vi "Simple Get Buffer.vi"(0 "remote file uri":string, 1 "username":string, 2 "password":string, 11 "error in (no error)":errorcluster) -> (4 "data":string, 15 "error out":errorcluster)   [LabVIEW 2017, in "NI_WebDAV.lvlib"]
doc: "Returns a file or multiple files or the raw binary contents of a file or multiple files from a remote WebDAV server or target. You must manually select the polymorphic instance you want to use."
uses:
  <vilib>/WebDAVClient/NI_WebDAV.lvlib
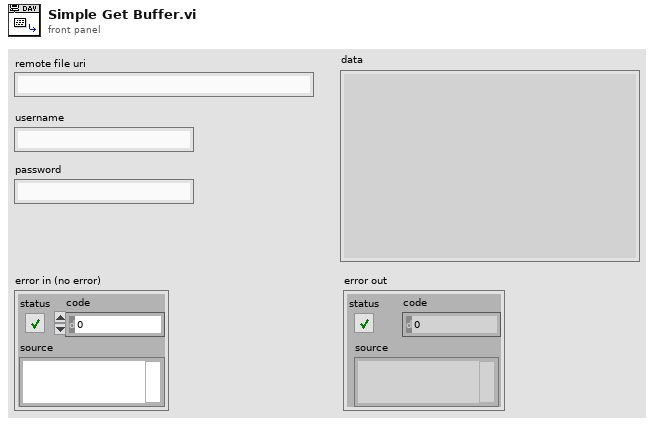
[diagram p1: front panel]
types:
  T1 = typedef "NI_WebDAV.lvlib/SessionHandle.ctl" = refnum<k1>
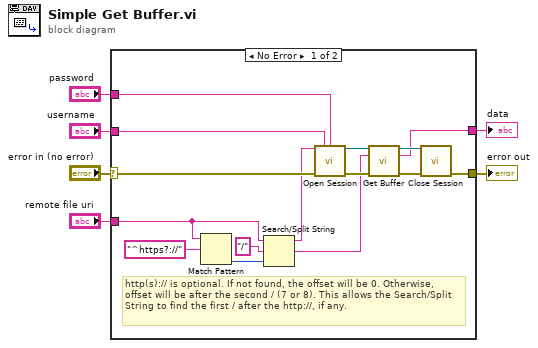
[diagram p0: block diagram]
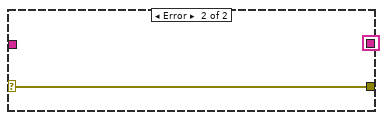
[diagram p2: hidden frame]
diagram:
  n1 = case shown="No Error" "error in (no error)" {
    selector: "error in (no error)" -> [w21 w23]
    tunnel: "username" -> [w20 _]
    tunnel: "password" -> [w19 _]
    tunnel: "remote file uri" -> [w9 _]
    tunnel: [w14 w23] -> w2
    tunnel: [w13 ""] -> w1
    frame No Error {
      # "http(s):// is optional. If not found, the offset will be 0. Otherwise, offset will be after the second / (7 or 8). This allows the Search/Split String to find the first / after the http://, if any."
      n2 = Match Pattern(string=w9, regular expression="^https?://") -> (offset past match=w12:i32)  [unwired: 1 in, 3 out]
      n3 = Search/Split String(string=w9, search string/char (-)="/", offset (0)=w12) -> (substring before match=w7:string, match + rest of string=w8:string)  [unwired: 1 out]
      n4 = call <vilib>:"Open Session.vi"("host uri prefix"=w7, "username"=w20, "password"=w19, "error in (no error)"=w21) -> ("session handle out"=w17:T1, "error out"=w18:errorcluster)  [unwired: 10 in]
      n5 = call <vilib>:"Get Buffer.vi"("session handle"=w17, "relative uri"=w8, "error in (no error)"=w18) -> ("session handle out"=w15:T1, "data"=w13:string, "error out"=w16:errorcluster)  [unwired: 10 in]
      n6 = call <vilib>:"Close Session.vi"("session handle"=w15, "error in (no error)"=w16) -> ("error out"=w14:errorcluster)  [unwired: 13 in]
    }
    frame Error {
    }
  }
  "error out" <- w2
  "data" <- w1
